vi "Configure simulated signals.vi"(9 "Q ramp length":i32, 10 "I ramp length":i32, 11 "FPGA VI Reference":T1) -> (3 "FPGA VI Reference out":T1)   [LabVIEW 2013]
uses:
  FPGAref.ctl
  <vilib>/rvi/interface/common/niFpgaWaitOnOcc.vi
  <vilib>/Utility/error.llb/Error Cluster From Error Code.vi
  <vilib>/rvi/errors/niLvFpgaAdjustHostInterfaceError.vi
  <vilib>/rvi/interface/nirviReadWriteControl/nirviReadWriteControl.xnode
  NiFpgaLv.dll
  <vilib>/rvi/interface/Simulation/niFpgaSimulationCallBeginRW.vi
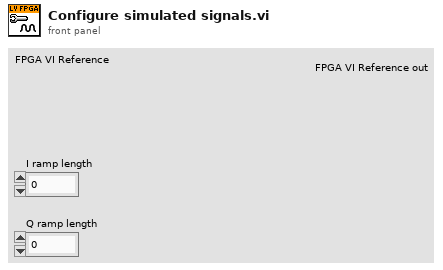
[diagram p1: front panel]
types:
  T1 = typedef "FPGAref.ctl" = refnum<k20>
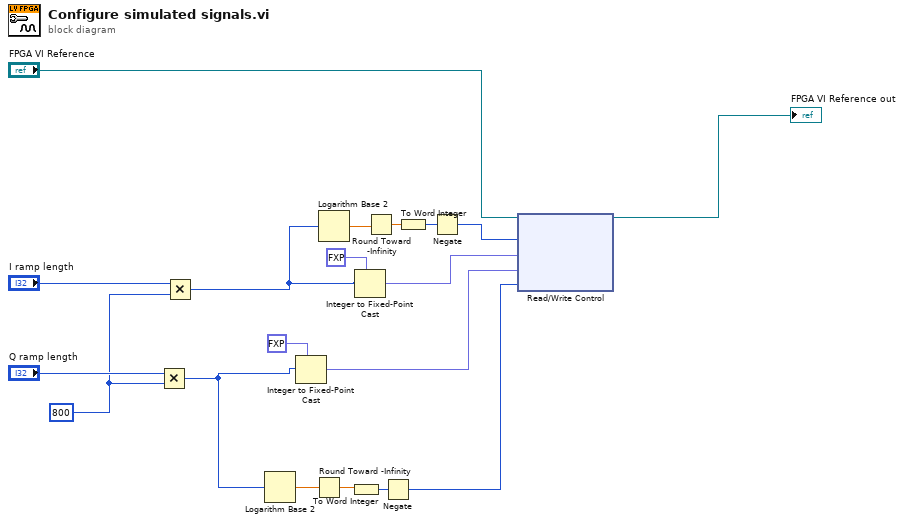
[diagram p0: block diagram]
diagram:
  w1 = 800 ("y")
  n1 = Multiply(x="Q ramp length", y=w1) -> (x*y=w4:i32)
  n2 = Multiply(x="I ramp length", y=w1) -> (x*y=w2:i32)
  n3 = Logarithm Base 2(1:w4) -> (0:w19:dbl)
  n4 = Integer to Fixed-Point Cast(fixed-point type=fxp<+/-,32,32> 0.0 ("I ramp length"), integer=w4) -> (fixed-point=w7:fxp<+/-,32,32>)
  n5 = Round Toward -Infinity(1:w19) -> (0:w18:dbl)
  n6 = Logarithm Base 2(1:w2) -> (0:w16:dbl)
  n7 = To Word Integer(number=w18) -> (16bit integer=w17:i16)
  n8 = Integer to Fixed-Point Cast(fixed-point type=fxp<+/-,32,32> 0.0 ("I ramp length"), integer=w2) -> (fixed-point=w8:fxp<+/-,32,32>)
  n9 = Round Toward -Infinity(1:w16) -> (0:w15:dbl)
  n10 = Negate(x=w17) -> (-x=w6:i16)
  n11 = To Word Integer(number=w15) -> (16bit integer=w14:i16)
  n12 = Negate(x=w14) -> (-x=w9:i16)
  n13 = xnode "Read/Write Control"("FPGA VI Reference In"="FPGA VI Reference", "I shift bits"=w9, "I ramp length"=w8, "Q ramp length"=w7, "Q shift bits"=w6) -> ("FPGA VI Reference Out"=→"FPGA VI Reference out":T1)  [unwired: 1 in, 1 out]
